vi "LFA_AcquireWithAutosave.vi"(8 "error in (no error)":errorcluster, 11 "LightField Automation in":refnum<class "LightField Automation.lvclass">) -> (0 "error out":errorcluster, 2 "Data":T1(array[cluster]), 3 "LightField Automation out":refnum<class "LightField Automation.lvclass">)   [LabVIEW 2018, in "LightField Automation.lvclass"]
uses:
  LightField Automation.lvclass
  LightField Automation.lvclass/LightField Automation.ctl
  C:/Users/xw9/Desktop/Turbulence program/SourceDistribution/PrincetonInstruments.LightFieldViewV3.dll
  PrincetonInstruments.LightFieldViewV3.dll
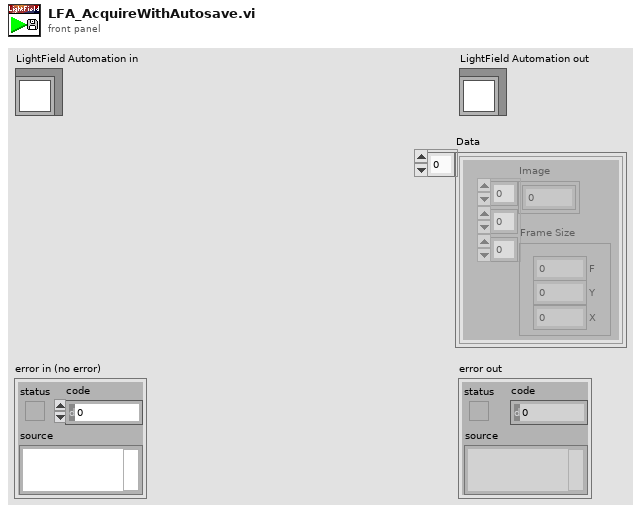
[diagram p1: front panel]
types:
  T1 = cluster{"Image":dbl[][][], "Frame Size":cluster{"F":i32, "Y":i32, "X":i32}}[]
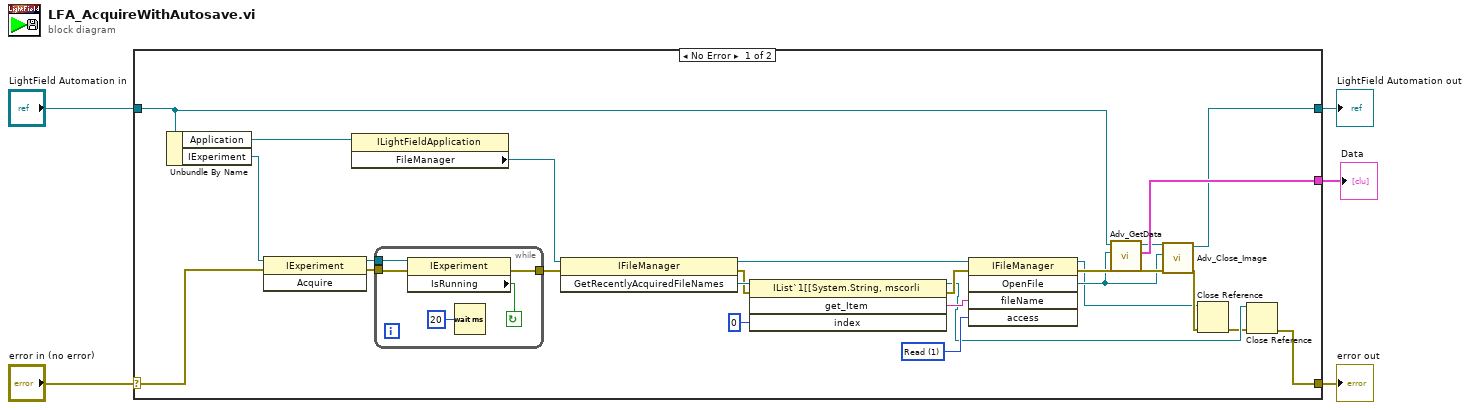
[diagram p0: block diagram]
diagram:
  n1 = case shown="No Error" "error in (no error)" {
    selector: "error in (no error)" -> [w31 w38]
    tunnel: [w14 w38] -> w4
    tunnel: [w10 w37] -> w2
    tunnel: "LightField Automation in" -> [w27 w37]
    tunnel: [w26 _] -> w1
    frame No Error {
      w16 = 1 items=["Read"=1, "Write"=2, "ReadWrite"=3] ("access")
      n2 = Unbundle By Name(w27) -> ("Application"=w25:refnum<k24>, "IExperiment"=w28:refnum<k24>)
      n3 = invoke class="IExperiment" method="Acquire"(reference=w28, error in=w31) -> (reference out=w29:refnum<k24>, error out=w30:errorcluster)  [unwired: 1 in, 1 out]
      n4 = property class="ILightFieldApplication"(reference=w25) -> ("FileManager"=w24:refnum<k24>)  [unwired: 1 in, 2 out]
      n5 = while {
        tunnel: w30 -> [w34]
        tunnel: [w33] -> w23
        tunnel: w29 -> [w32]
        stop <- w36 continue-if-true
        n6 = property class="IExperiment"(reference=w32, error in=w34) -> (error out=w33:errorcluster, "IsRunning"=w36:bool)  [unwired: 1 out]
        n7 = Wait (ms)(milliseconds to wait=u32 20) -> ()  [unwired: 1 out]
      }
      n8 = invoke class="IFileManager" method="GetRecentlyAcquiredFileNames"(reference=w24, error in=w23) -> (reference out=w18:refnum<k24>, error out=w21:errorcluster, "GetRecentlyAcquiredFileNames"=w22:refnum<k24>)  [unwired: 1 in]
      n9 = invoke class="IList`1[[System.String, mscorli" method="get_Item"(reference=w22, error in=w21, "index"=0) -> (reference out=w13:refnum<k24>, error out=w19:errorcluster, "get_Item"=w17:string)  [unwired: 1 in, 1 out]
      n10 = invoke class="IFileManager" method="OpenFile"(reference=w18, error in=w19, "fileName"=w17, "access"=w16) -> (reference out=w6:refnum<k24>, error out=w15:errorcluster, "OpenFile"=w7:refnum<k24>)  [unwired: 1 in, 2 out]
      n11 = call "Adv_GetData.vi"("error in (no error)"=w15, "IImageDataSet"=w7, "LightField Automation in"=w27) -> ("error out"=w12:errorcluster, "Data"=w26:T1, "LightField Automation out"=w11:refnum<class "LightField Automation.lvclass">)  [unwired: 6 in]
      n12 = call "Adv_Close_Image.vi"("error in (no error)"=w12, "ImageDataSet"=w7, "LightField Automation in"=w11) -> ("error out"=w8:errorcluster, "LightField Automation out"=w10:refnum<class "LightField Automation.lvclass">)  [unwired: 7 in]
      n13 = Close Reference(reference=w6, error in (no error)=w8) -> (error out=w9:errorcluster)
      n14 = Close Reference(reference=w13, error in (no error)=w9) -> (error out=w14:errorcluster)
    }
    frame Error {
    }
  }
  "error out" <- w4
  "LightField Automation out" <- w2
  "Data" <- w1
